vi "ROI entry screen-LBox select plans for copy.vi"() -> ()   [LabVIEW 2020]
panel:
  in  "?":i32(listbox)
  in  "Value":i32
  in  "Add 2":bool
  in  "Add":bool
  in  "Selected ROI plane":i32(listbox)
  in  "To Plane":u16(ring)
  in  "From Plane":u16(ring)
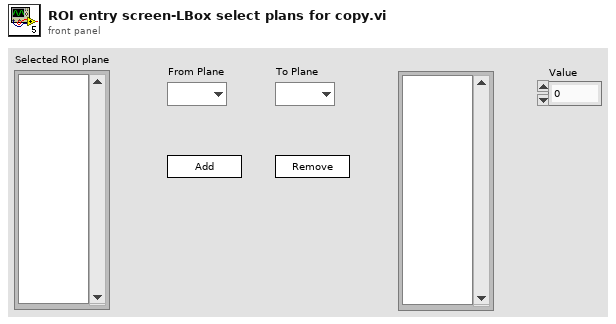
[diagram p1: front panel]
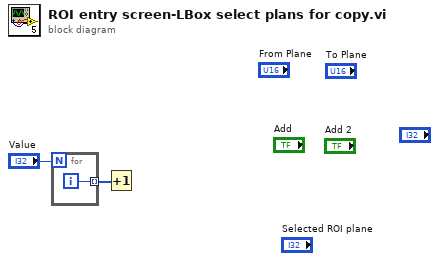
[diagram p0: block diagram]
diagram:
  n1 = for {
    N: "Value" -> [_]
    tunnel: [w3] -> w1 mode=indexing
    i -> [w3]
  }
  n2 = Increment(x=w1) -> ()  [unwired: 1 out]
